vi "StellarNet Init & Count.vi"(8 "error in (no error)":errorcluster, 11 "reference":path) -> (0 "error out":errorcluster, 3 "Number of Channels":i32)   [LabVIEW 2023]
panel:
  # "This subVI initializes the .dll and returns the number of attached spectrometers found by the .dll"
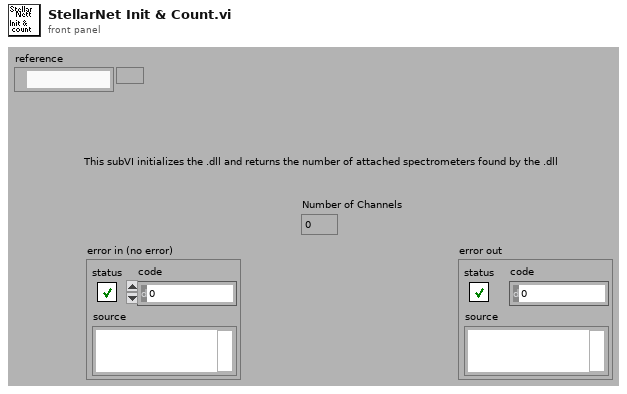
[diagram p1: front panel]
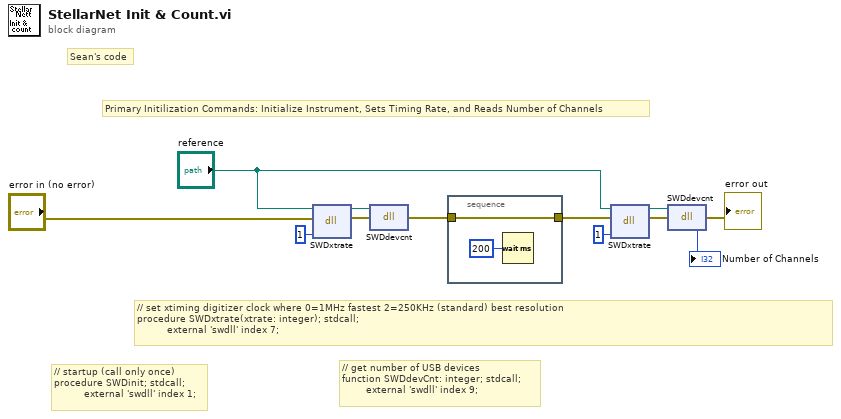
[diagram p0: block diagram]
diagram:
  # "Sean's code"
  # "// get number of USB devices\nfunction SWDdevCnt: integer; stdcall;\n        external 'swdll' index 9;"
  # "// set xtiming digitizer clock where 0=1MHz fastest 2=250KHz (standard) best resolution \nprocedure SWDxtrate(xtrate: integer); stdcall;\n          external 'swdll' index 7;"
  # "// startup (call only once)\nprocedure SWDinit; stdcall;\n          external 'swdll' index 1;"
  # "Primary Initilization Commands: Initialize Instrument, Sets Timing Rate, and Reads Number of Channels"
  n1 = dll-call lib="C:/Program Files/StellarNet/SpectraWiz/swdll.dll" fn="SWDxtrate" label="xtrate"(path in="reference", error in="error in (no error)", "xtrate"=1) -> (path out=w9:path, error out=w11:errorcluster)  [unwired: 3 in]
  n2 = dll-call lib="C:/Program Files/StellarNet/SpectraWiz/swdll.dll" fn="SWDdevcnt"(path in=w9, error in=w11) -> (error out=w8:errorcluster)  [unwired: 2 in, 1 out]
  n3 = stacked-sequence {
    tunnel: w8 -> [w13]
    tunnel: [w13] -> w4
    frame #0 {
      n4 = Wait (ms)(milliseconds to wait=u32 200) -> ()  [unwired: 1 out]
    }
  }
  n5 = dll-call lib="C:/Program Files/StellarNet/SpectraWiz/swdll.dll" fn="SWDxtrate" label="xtrate"(path in="reference", error in=w4, "xtrate"=1) -> (path out=w7:path, error out=w6:errorcluster)  [unwired: 3 in]
  n6 = dll-call lib="C:/Program Files/StellarNet/SpectraWiz/swdll.dll" fn="SWDdevcnt"(path in=w7, error in=w6) -> (error out=→"error out":errorcluster, "NumChan"=→"Number of Channels":i32)  [unwired: 1 in, 1 out]
